vi "meth.Table2Cluster.vi"(0 "class.GLue in":refnum<class "class.GLue.lvclass">, 11 "error in":errorcluster) -> (4 "class.GLue out":refnum<class "class.GLue.lvclass">, 8 "Cluster":variant, 15 "error out":errorcluster)   [LabVIEW 2014, in "GLue.lvlib" / "class.GLue.lvclass"]
uses:
  class.GLue.lvclass
  class.GLue.lvclass/class.GLue.ctl
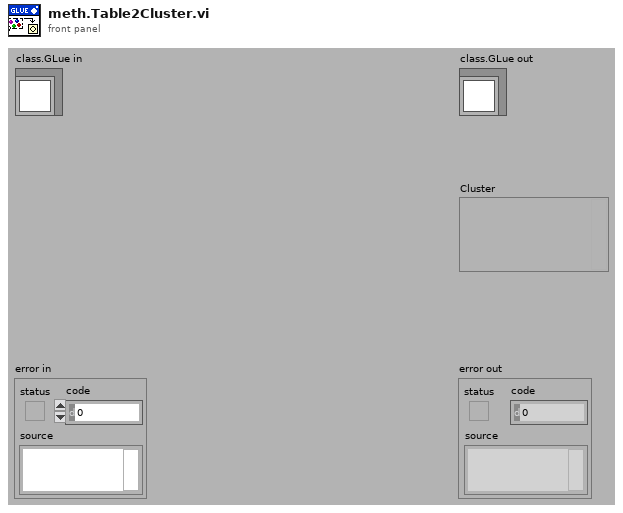
[diagram p1: front panel]
types:
  T1 = typedef "GLue.lvlib/class.GLue.lvclass/typedef.Types.ctl" = enum16{"Nil", "Bool", "LightUserData", "Number", "String", "Table", "Function", "UserData", "Thread"}
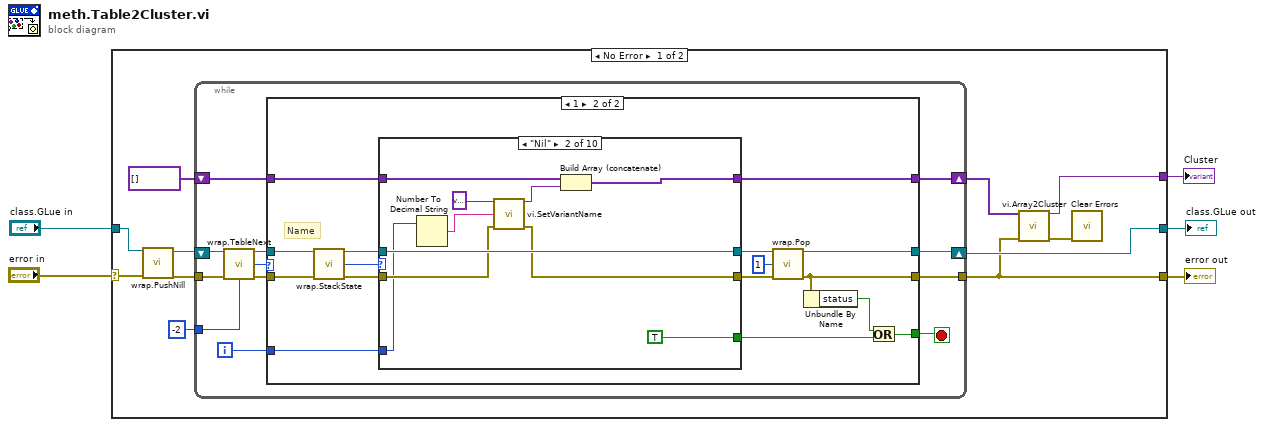
[diagram p0: block diagram]
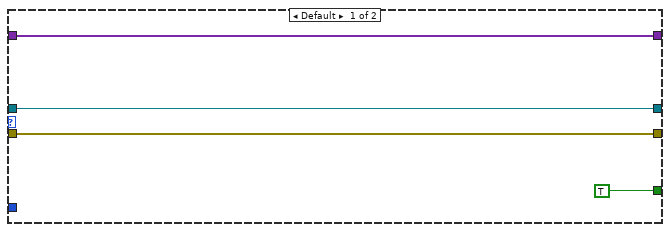
[diagram p2: hidden frame]
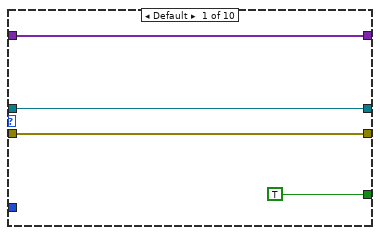
[diagram p3: hidden frame]
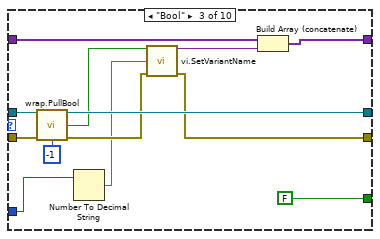
[diagram p4: hidden frame]
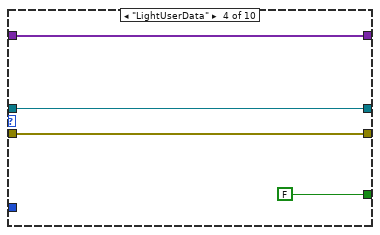
[diagram p5: hidden frame]
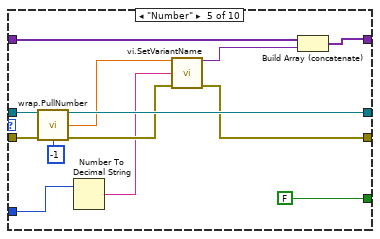
[diagram p6: hidden frame]
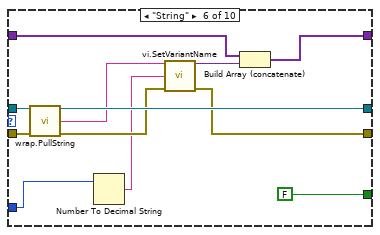
[diagram p7: hidden frame]
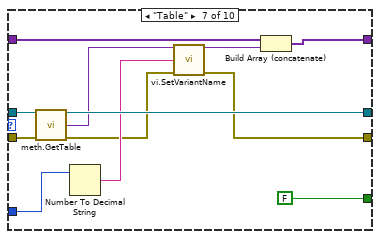
[diagram p8: hidden frame]
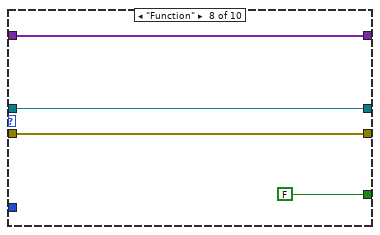
[diagram p9: hidden frame]
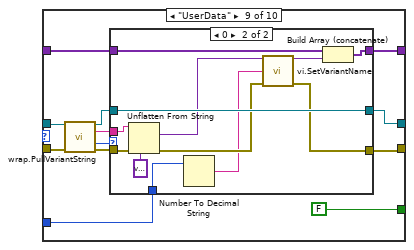
[diagram p10: hidden frame]
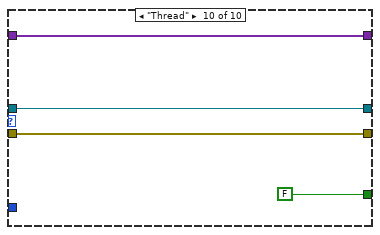
[diagram p12: hidden frame]
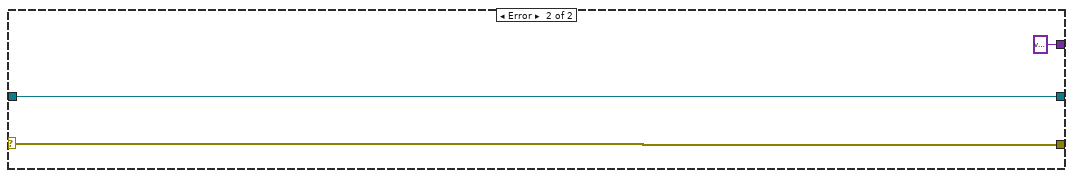
[diagram p13: hidden frame]
diagram:
  n1 = case shown="No Error" "error in" {
    selector: "error in" -> [w11 w154]
    tunnel: [w6 w154] -> w4
    tunnel: [w7 w153] -> w2
    tunnel: "class.GLue in" -> [w9 w153]
    tunnel: [w10 variant ("Cluster")] -> w1
    frame No Error {
      n2 = call "wrap.PushNill.vi"("class.GLue in"=w9, "error in (no error)"=w11) -> ("class.GLue out"=w13:refnum<class "class.GLue.lvclass">, "error out"=w12:errorcluster)  [unwired: 12 in]
      n3 = while {
        tunnel: -2 ("Numeric") -> [w23]
        tunnel: w12 -> [w28]
        shift-right: [w19] -> w15
        shift-left: variant[] [] ("Table") -> [w24]
        shift-right: [w21] -> w7
        shift-left: w13 -> [w27]
        tunnel: [w20] -> w6
        i -> [w17]
        stop <- w18 stop-if-true
        n4 = call "wrap.TableNext.vi"("class.GLue in"=w27, "error in (no error)"=w28, "Index"=w23) -> ("class.GLue out"=w25:refnum<class "class.GLue.lvclass">, "Return"=w22:i32, "error out"=w26:errorcluster)  [unwired: 10 in]
        n5 = case shown="1" w22 {
          tunnel: w26 -> [w31 w40]
          tunnel: w25 -> [w30 w39]
          tunnel: [TRUE w36] -> w18
          tunnel: w24 -> [w29 w45]
          tunnel: [w30 w42] -> w21
          tunnel: [w31 w37] -> w20
          tunnel: [w29 w41] -> w19
          tunnel: w17 -> [_ w33]
          frame Default {
          }
          frame 1 {
            # "Name"
            n6 = call "wrap.StackState.vi"("class.GLue in"=w39, "error in (no error)"=w40) -> ("class.GLue out"=w47:refnum<class "class.GLue.lvclass">, "TopType"=w48:T1, "error out"=w46:errorcluster)  [unwired: 10 in, 1 out]
            n7 = case shown="\"Nil\"" w48 {
              tunnel: w47 -> [w51 w62 w75 w78 w90 w104 w116 w119 w130 w150]
              tunnel: w46 -> [w52 w56 w74 w77 w89 w103 w114 w118 w131 w149]
              tunnel: w45 -> [w50 w60 w71 w79 w92 w102 w113 w120 w123 w151]
              tunnel: [w52 w55 w65 w77 w80 w95 w105 w118 w125 w149] -> w44
              tunnel: [w51 w62 w72 w78 w88 w100 w115 w119 w126 w150] -> w43
              tunnel: [w50 w59 w70 w79 w91 w101 w112 w120 w122 w151] -> w41
              tunnel: [TRUE TRUE FALSE FALSE FALSE FALSE FALSE FALSE FALSE FALSE] -> w34
              tunnel: w33 -> [_ w54 w64 _ w85 w94 w108 _ w121 _]
              frame Default {
              }
              frame "Nil" {
                n8 = Number To Decimal String(number=w54) -> (decimal integer string=w53:string)  [unwired: 1 in]
                n9 = call "vi.SetVariantName.vi"("Variant in"=variant ("variant"), "Name"=w53, "error in"=w56) -> ("Named Variant"=w57:variant, "error out"=w55:errorcluster)  [unwired: 11 in]
                n10 = Build Array (concatenate)(w60, w57) -> (w59:variant[])
              }
              frame "Bool" {
                n11 = call "wrap.PullBool.vi"("class.GLue in"=w75, "error in (no error)"=w74, "Index"=-1) -> ("class.GLue out"=w72:refnum<class "class.GLue.lvclass">, "Boolean"=w68:bool, "error out"=w66:errorcluster)  [unwired: 10 in]
                n12 = Number To Decimal String(number=w64) -> (decimal integer string=w63:string)  [unwired: 1 in]
                n13 = call "vi.SetVariantName.vi"("Variant in"=w68, "Name"=w63, "error in"=w66) -> ("Named Variant"=w67:variant, "error out"=w65:errorcluster)  [unwired: 11 in]
                n14 = Build Array (concatenate)(w71, w67) -> (w70:variant[])
              }
              frame "LightUserData" {
              }
              frame "Number" {
                n15 = call "wrap.PullNumber.vi"("class.GLue in"=w90, "error in (no error)"=w89, "Index"=-1) -> ("class.GLue out"=w88:refnum<class "class.GLue.lvclass">, "Number"=w82:dbl, "error out"=w84:errorcluster)  [unwired: 10 in]
                n16 = Number To Decimal String(number=w85) -> (decimal integer string=w83:string)  [unwired: 1 in]
                n17 = call "vi.SetVariantName.vi"("Variant in"=w82, "Name"=w83, "error in"=w84) -> ("Named Variant"=w81:variant, "error out"=w80:errorcluster)  [unwired: 11 in]
                n18 = Build Array (concatenate)(w92, w81) -> (w91:variant[])
              }
              frame "String" {
                n19 = call "wrap.PullString.vi"("class.GLue in"=w104, "error in (no error)"=w103) -> ("class.GLue out"=w100:refnum<class "class.GLue.lvclass">, "String"=w98:string, "error out"=w96:errorcluster)  [unwired: 11 in]
                n20 = Number To Decimal String(number=w94) -> (decimal integer string=w93:string)  [unwired: 1 in]
                n21 = call "vi.SetVariantName.vi"("Variant in"=w98, "Name"=w93, "error in"=w96) -> ("Named Variant"=w97:variant, "error out"=w95:errorcluster)  [unwired: 11 in]
                n22 = Build Array (concatenate)(w102, w97) -> (w101:variant[])
              }
              frame "Table" {
                n23 = call "meth.GetTable.vi"("class.GLue in"=w116, "error in (no error)"=w114) -> ("class.GLue out"=w115:refnum<class "class.GLue.lvclass">, "Table"=w110:variant, "error out"=w106:errorcluster)  [unwired: 11 in]
                n24 = Number To Decimal String(number=w108) -> (decimal integer string=w107:string)  [unwired: 1 in]
                n25 = call "vi.SetVariantName.vi"("Variant in"=w110, "Name"=w107, "error in"=w106) -> ("Named Variant"=w109:variant, "error out"=w105:errorcluster)  [unwired: 11 in]
                n26 = Build Array (concatenate)(w113, w109) -> (w112:variant[])
              }
              frame "Function" {
              }
              frame "UserData" {
                n27 = call "wrap.PullVariantString.vi"("class.GLue in"=w130, "error in (no error)"=w131) -> ("class.GLue out"=w127:refnum<class "class.GLue.lvclass">, "VarString"=w124:string, "Return"=w128:i32, "error out"=w129:errorcluster)  [unwired: 10 in]
                n28 = case shown="0" w128 {
                  tunnel: w129 -> [w133 w147]
                  tunnel: w127 -> [w134 w146]
                  tunnel: [w134 w146] -> w126
                  tunnel: [w133 w138] -> w125
                  tunnel: w124 -> [_ w144]
                  tunnel: w123 -> [w135 w143]
                  tunnel: [w135 w142] -> w122
                  tunnel: w121 -> [_ w137]
                  frame Default {
                  }
                  frame 0 {
                    n29 = Unflatten From String(type=variant ("Cluster"), binary string=w144, error in (no error)=w147) -> (value=w141:variant, error out=w139:errorcluster)  [unwired: 2 in, 1 out]
                    n30 = Number To Decimal String(number=w137) -> (decimal integer string=w136:string)  [unwired: 1 in]
                    n31 = call "vi.SetVariantName.vi"("Variant in"=w141, "Name"=w136, "error in"=w139) -> ("Named Variant"=w140:variant, "error out"=w138:errorcluster)  [unwired: 11 in]
                    n32 = Build Array (concatenate)(w143, w140) -> (w142:variant[])
                  }
                }
              }
              frame "Thread" {
              }
            }
            n33 = call "wrap.Pop.vi"("class.GLue in"=w43, "Num"=1, "error in (no error)"=w44) -> ("class.GLue out"=w42:refnum<class "class.GLue.lvclass">, "error out"=w37:errorcluster)  [unwired: 11 in]
            n34 = Unbundle By Name(w37) -> ("status"=w35:bool)
            n35 = Or(x=w35, y=w34) -> (x .or. y?=w36:bool)
          }
        }
      }
      n36 = call "vi.Array2Cluster.vi"("Array"=w15, "error in (no error)"=w6) -> ("Cluster"=w10:variant, "error out"=w16:errorcluster)  [unwired: 12 in]
      n37 = call <vilib>:"Clear Errors.vi"("error in (no error)"=w16) -> ()  [unwired: 5 in, 2 out]
    }
    frame Error {
    }
  }
  "error out" <- w4
  "class.GLue out" <- w2
  "Cluster" <- w1
